vi "Get Devices And Channels.vi"() -> ()   [LabVIEW 2020]
uses:
  <resource>/objmgr/daqmx.rc
panel:
  out "AI.PhysicalChans":tag[](array[tag])
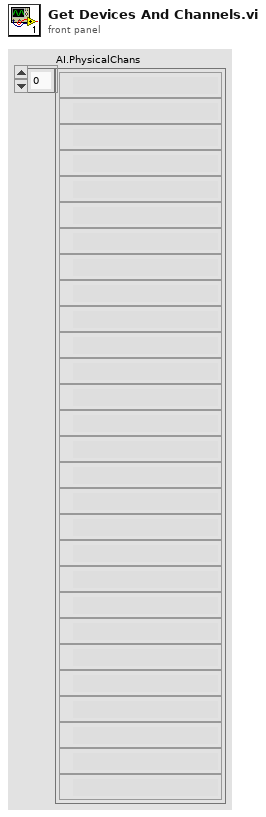
[diagram p1: front panel]
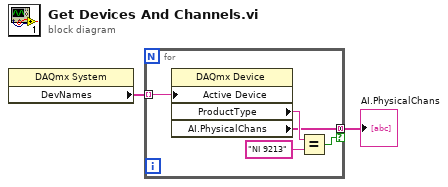
[diagram p0: block diagram]
diagram:
  n1 = property class="DAQmx System"() -> ("DevNames"=w2:tag[])  [unwired: 2 in, 2 out]
  n2 = for {
    tunnel: w2 -> [w7] mode=indexing
    tunnel: [w4] -> w1 mode=concatenating if=w3
    n3 = property class="DAQmx Device"("Active Device"=w7) -> ("ProductType"=w5:string, "AI.PhysicalChans"=w4:tag[])  [unwired: 2 in, 2 out]
    n4 = Equal?(x=w5, y="NI 9213") -> (x = y?=w3:bool)
  }
  "AI.PhysicalChans" <- w1
